vi "MGI Centered Weighted Moving Average.vi"(8 "Array In[]":dbl[](array[numeric]), 9 "Weights[]":i32[](array[numeric]), 10 "Weighting (Equal)":T1(ring), 11 "Size (should be odd)":u32) -> (0 "Array Out[]":dbl[](array[numeric]), 2 "Average":dbl)   [LabVIEW 2016]
doc: "Performs a centered weighted moving average on an array according to the size and weighting parameters.\n\nAuthored by Robert C. Mortensen\nsupport@mooregoodideas.com\nwww.mooregoodideas.com\n\nCopyright (c) 2010, Moore Good Ideas, Inc.\n\nAll rights reserved.\n\nRedistribution and use in source and binary forms, with or without modification, are permitted provided that the following conditions are met:\n\n * Redistributions of source code must retain the above copyright notice, this list of conditions and the following disclaimer.\n * Redistributions in binary form must reproduce the above copyright notice, this list of conditions and the following disclaimer in the documentation and/or other materials provided with the distribution.\n * Neither the name of Moore Good Ideas, Inc. nor the names of its contributors may be used to endorse or promote products derived from this software without specific prior written permission.\n\nTHIS SOFTWARE IS PROVIDED BY THE COPYRIGHT HOLDERS AND CONTRIBUTORS \"AS IS\" AND ANY EXPRESS OR IMPLIED WARRANTIES, INCLUDING, BUT NOT LIMITED TO, THE IMPLIED WARRANTIES OF MERCHANTABILITY AND FITNESS FOR A PARTICULAR PURPOSE ARE DISCLAIMED. IN NO EVENT SHALL THE COPYRIGHT OWNER OR CONTRIBUTORS BE LIABLE FOR ANY DIRECT, INDIRECT, INCIDENTAL, SPECIAL, EXEMPLARY, OR CONSEQUENTIAL DAMAGES (INCLUDING, BUT NOT LIMITED TO, PROCUREMENT OF SUBSTITUTE GOODS OR SERVICES; LOSS OF USE, DATA, OR PROFITS; OR BUSINESS INTERRUPTION) HOWEVER CAUSED AND ON ANY THEORY OF LIABILITY, WHETHER IN CONTRACT, STRICT LIABILITY, OR TORT (INCLUDING NEGLIGENCE OR OTHERWISE) ARISING IN ANY WAY OUT OF THE USE OF THIS SOFTWARE, EVEN IF ADVISED OF THE POSSIBILITY OF SUCH DAMAGE."
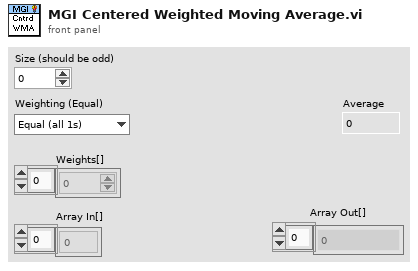
[diagram p1: front panel]
types:
  T1 = enum16{"Equal (all 1s)", "Equal Step (1 2 3 4 3 2 1)", "Custom (Use Terminal)"}
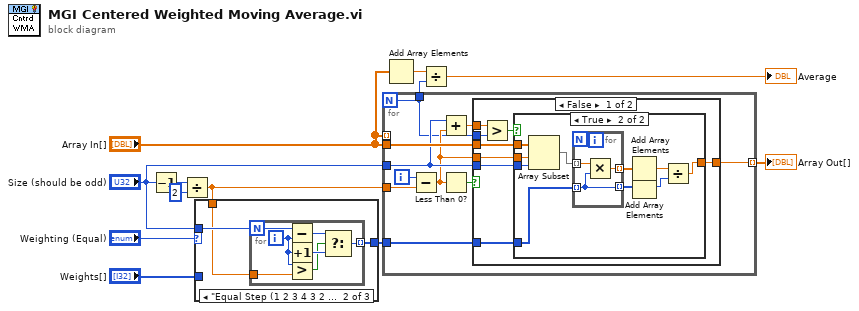
[diagram p0: block diagram]
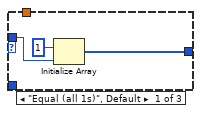
[diagram p2: hidden frame]
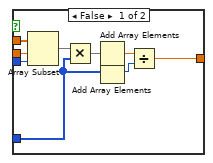
[diagram p4: hidden frame]
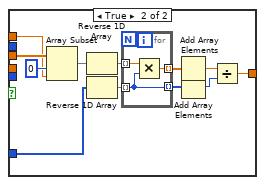
[diagram p5: hidden frame]
diagram:
  n1 = Decrement(x="Size (should be odd)") -> (x-1=w5:u32)
  n2 = Divide(x=w5, y=2) -> (x/y=w10:dbl)
  n3 = case shown="\"Equal Step (1 2 3 4 3 2 1)\"" "Weighting (Equal)" {
    tunnel: "Size (should be odd)" -> [w15 w18 _]
    tunnel: w10 -> [_ w17 _]
    tunnel: [w13 w16 w26] -> w8
    tunnel: "Weights[]" -> [_ _ w26]
    frame "Equal (all 1s)", Default {
      n4 = Initialize Array(1 ("element"), w15) -> (w13:i32[])
    }
    frame "Equal Step (1 2 3 4 3 2 1)" {
      n5 = for {
        N: w18 -> [w25]
        tunnel: w17 -> [w22]
        tunnel: [w19] -> w16 mode=indexing
        i -> [w21]
        n6 = Subtract(x=w25, y=w21) -> (x-y=w23:i32)
        n7 = Increment(x=w21) -> (x+1=w24:i32)
        n8 = Greater?(x=w21, y=w22) -> (0:w20:bool)
        n9 = Select(t=w23, s=w20, f=w24) -> (s? t:f=w19:i32)
      }
    }
    frame "Custom (Use Terminal)" {
    }
  }
  n10 = for {
    N -> [w27]
    tunnel: "Array In[]" -> [w36]
    tunnel: "Size (should be odd)" -> [w32]
    tunnel: "Array In[]" -> [_] mode=indexing
    tunnel: w10 -> [w28]
    tunnel: w8 -> [w30]
    tunnel: [w29] -> w9 mode=indexing
    tunnel: [w27] -> w2
    i -> [w35]
    n11 = Subtract(x=w35, y=w28) -> (x-y=w31:dbl)
    n12 = Add(x=w32, y=w31) -> (x+y=w33:dbl)
    n13 = Less Than 0?(x=w31) -> (x < 0?=w34:bool)
    n14 = case shown="False" w34 {
      tunnel: w36 -> [w44 w78]
      tunnel: w33 -> [w43 w76]
      tunnel: w27 -> [w42 _]
      tunnel: w32 -> [w40 _]
      tunnel: w31 -> [w39 _]
      tunnel: w30 -> [w38 w74]
      tunnel: [w37 w67] -> w29
      frame False {
        n15 = Greater?(x=w43, y=w42) -> (0:w41:bool)
        n16 = case shown="True" w41 {
          tunnel: w44 -> [w53 w63]
          tunnel: w40 -> [w52 w62]
          tunnel: w39 -> [w51 w61]
          tunnel: w38 -> [w46 w55]
          tunnel: [w45 w54] -> w37
          frame False {
            n17 = Array Subset(array=w53, index=w51, length=w52) -> (w50:dbl[])
            n18 = Multiply(x=w50, y=w46) -> (x*y=w47:dbl[])
            n19 = Add Array Elements(numeric array=w47) -> (sum=w48:dbl)
            n20 = Add Array Elements(numeric array=w46) -> (sum=w49:i32)
            n21 = Divide(x=w48, y=w49) -> (x/y=w45:dbl)
          }
          frame True {
            n22 = Array Subset(array=w63, index=w61, length=w62) -> (w56:dbl[])
            n23 = for {
              tunnel: w56 -> [w66] mode=indexing
              tunnel: w55 -> [w65] mode=indexing
              tunnel: [w65] -> w58 mode=indexing
              tunnel: [w64] -> w57 mode=indexing
              n24 = Multiply(x=w66, y=w65) -> (x*y=w64:dbl)
            }
            n25 = Add Array Elements(numeric array=w57) -> (sum=w60:dbl)
            n26 = Add Array Elements(numeric array=w58) -> (sum=w59:i32)
            n27 = Divide(x=w60, y=w59) -> (x/y=w54:dbl)
          }
        }
      }
      frame True {
        n28 = Array Subset(array=w78, index=0, length=w76) -> (w75:dbl[])
        n29 = Reverse 1D Array(array=w75) -> (reversed array=w73:dbl[])
        n30 = Reverse 1D Array(array=w74) -> (reversed array=w72:i32[])
        n31 = for {
          tunnel: w73 -> [w81] mode=indexing
          tunnel: w72 -> [w80] mode=indexing
          tunnel: [w80] -> w70 mode=indexing
          tunnel: [w79] -> w71 mode=indexing
          n32 = Multiply(x=w81, y=w80) -> (x*y=w79:dbl)
        }
        n33 = Add Array Elements(numeric array=w71) -> (sum=w68:dbl)
        n34 = Add Array Elements(numeric array=w70) -> (sum=w69:i32)
        n35 = Divide(x=w68, y=w69) -> (x/y=w67:dbl)
      }
    }
  }
  "Array Out[]" <- w9
  n36 = Add Array Elements(numeric array="Array In[]") -> (sum=w3:dbl)
  n37 = Divide(x=w3, y=w2) -> (x/y=→"Average":dbl)
